vi "Locate and Read Data Socket.vi"(8 "error in":errorcluster, 9 "Browser Start URL":string="dstp://cryogenicsystem", 10 "Browse for URL":bool=TRUE, 11 "DataSocket URL":string="dstp://cryogenicsystem/sensor a") -> (0 "error out":errorcluster, 3 "DataSocket data":variant)   [LabVIEW 2021]
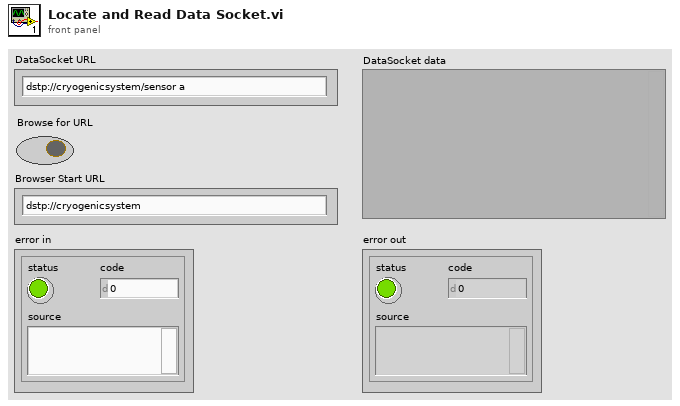
[diagram p1: front panel]
types:
  T1 = enum16{"Read", "Write", "ReadWrite", "BufferedRead", "BufferedReadWrite"}
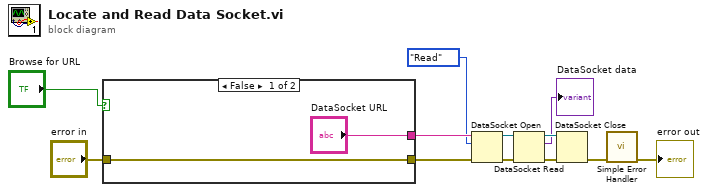
[diagram p0: block diagram]
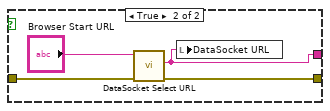
[diagram p2: hidden frame]
diagram:
  n1 = case shown="False" "Browse for URL" {
    tunnel: ["DataSocket URL" w17] -> w12
    tunnel: [w14 w18] -> w9
    tunnel: "error in" -> [w14 w16]
    frame False {
    }
    frame True {
      n2 = call <vilib>:"DataSocket Select URL.vi"("error in (no error)"=w16, "StartURL (empty)"="Browser Start URL") -> ("error out"=w18:errorcluster, "URL"=w17:string)  [unwired: 7 in, 1 out]
      n3 = local write "DataSocket URL"(w17) -> ()
    }
  }
  n4 = DataSocket Open(8:w9, 10:T1."Read" ("mode"), 11:w12) -> (0:w8:errorcluster, 3:w11:refnum<k13>)  [unwired: 1 in]
  n5 = DataSocket Read(8:w8, 11:w11) -> (0:w7:errorcluster, 2:→"DataSocket data":variant, 3:w10:refnum<k13>)  [unwired: 3 in, 4 out]
  n6 = DataSocket Close(8:w7, 11:w10) -> (0:w6:errorcluster)  [unwired: 1 in, 1 out]
  n7 = call <vilib>:"Simple Error Handler.vi"("error in (no error)"=w6) -> ("error out"=→"error out":errorcluster)  [unwired: 4 in, 4 out]
